vi "CT-Compute Max Level.vi"(0 "HCT Runtime":T3, 9 "Level":T1, 11 "error in (no error)":errorcluster) -> (6 "Max Level":dbl, 10 "Level out":T1, 15 "error out":errorcluster)   [LabVIEW 2020]
uses:
  CT-Runtime Data.ctl
  Controls/Level XCtl/Level Data.ctl
  Controls/Level XCtl/Level Units.ctl
  Utility VIs/Math VIs/Linear to dB (scalar).vi
  PXI DAQ VIs/DAQ Engine VIs/PXI Globals.vi
  Controls/Level XCtl/Level XCtl.xctl
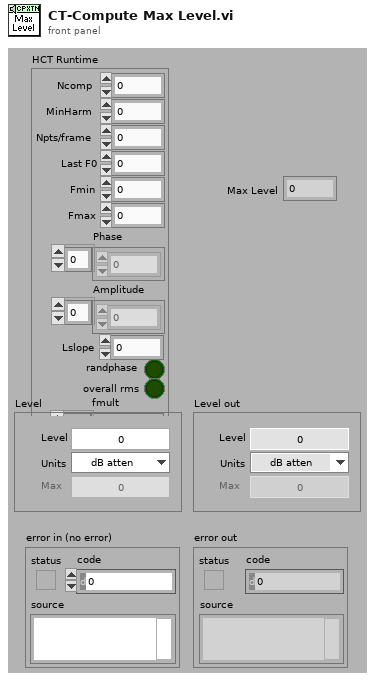
[diagram p1: front panel]
types:
  T1 = typedef "Level XCtl.xctl/Level Data.ctl" = cluster{"Level":dbl, "Units":T2, "Max":dbl, "Multiplier":dbl, "Cal File":path, "Cal":cluster{"Freq (Hz)":dbl[], "Mag (dB SPL)":dbl[], "Phase (deg)":dbl[]}}
  T2 = typedef "Level Units.ctl" = enum16{"dB atten", "dB SPL", "dB re 1 Vrms", "dB V/Hz½", "mW", "dB HL", "Volts", "dB mW"}
  T3 = typedef "CT-Runtime Data.ctl" = cluster{"Ncomp":i32, "MinHarm":i32, "Phase":dbl[], "Amplitude":dbl[], "Npts/frame":i32, "Last F0":dbl, "Fmin":dbl, "Fmax":dbl, "Lslope":dbl, "randphase":bool, "overall rms":bool, "fmult":dbl[], "jittered":bool}
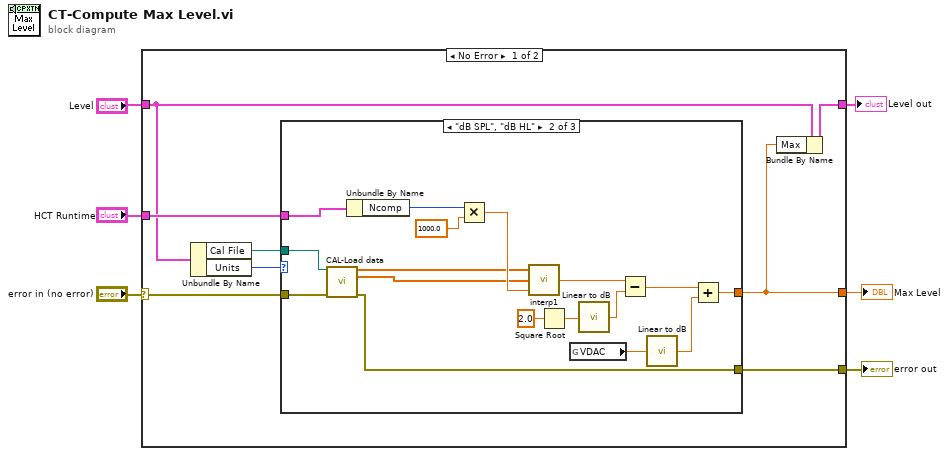
[diagram p0: block diagram]
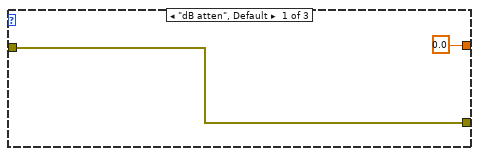
[diagram p2: hidden frame]
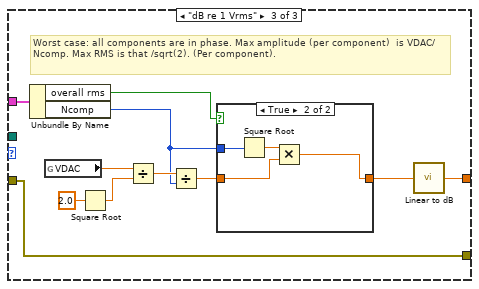
[diagram p3: hidden frame]
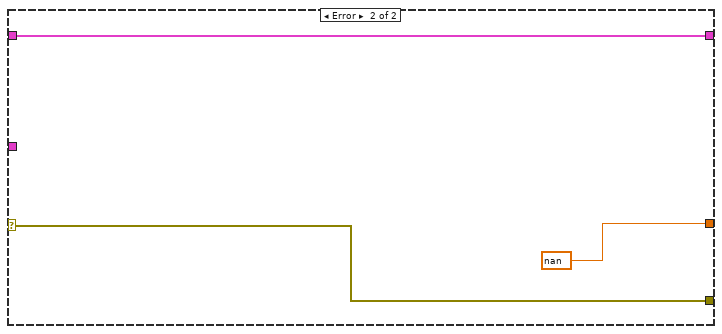
[diagram p5: hidden frame]
diagram:
  n1 = case shown="No Error" "error in (no error)" {
    selector: "error in (no error)" -> [w14 w52]
    tunnel: "Level" -> [w11 w50]
    tunnel: "HCT Runtime" -> [w13 _]
    tunnel: [w12 w52] -> w5
    tunnel: [w10 nan ("Reference Level")] -> w2
    tunnel: [w9 w50] -> w1
    frame No Error {
      n2 = Unbundle By Name(w11) -> ("Cal File"=w8:path, "Units"=w7:T2)
      n3 = case shown="\"dB SPL\", \"dB HL\"" w7 {
        tunnel: w14 -> [w15 w33 w44]
        tunnel: w13 -> [_ w24 w40]
        tunnel: [0.0 ("Reference Level") w31 w34] -> w10
        tunnel: [w15 w20 w44] -> w12
        tunnel: w8 -> [_ w19 _]
        frame "dB atten", Default {
        }
        frame "dB SPL", "dB HL" {
          n4 = call "CAL-Load data.vi"("user path"=w19, "error in (no error)"=w33) -> ("Frequency (Hz)"=w18:dbl[], "Mag"=w17:dbl[], "error out"=w20:errorcluster)  [unwired: 6 in, 5 out]
          n5 = Unbundle By Name(w24) -> ("Ncomp"=w29:i32)
          n6 = Multiply(x=w29, y=1000.0) -> (x*y=w27:dbl)
          n7 = call "interp1.vi"("X"=w18, "Y"=w17, "U"=w27) -> ("V"=w25:dbl)  [unwired: 2 in]
          n8 = Square Root(x=2.0 ("y")) -> (sqrt(x)=w23:dbl)
          n9 = global read "PXI Globals.vi" "VDAC"() -> (w32:dbl)
          n10 = call-poly "Linear to dB.vi"("Linear"=w23) -> ("dB"=w22:dbl)
          n11 = Subtract(x=w25, y=w22) -> (x-y=w21:dbl)
          n12 = call-poly "Linear to dB.vi"("Linear"=w32) -> ("dB"=w30:dbl)
          n13 = Add(x=w21, y=w30) -> (x+y=w31:dbl)
        }
        frame "dB re 1 Vrms" {
          # "Worst case: all components are in phase. Max amplitude (per component)  is VDAC/Ncomp. Max RMS is that /sqrt(2). (Per component)."
          n14 = Unbundle By Name(w40) -> ("overall rms"=w36:bool, "Ncomp"=w38:i32)
          n15 = global read "PXI Globals.vi" "VDAC"() -> (w41:dbl)
          n16 = Square Root(x=2.0 ("y")) -> (sqrt(x)=w42:dbl)
          n17 = Divide(x=w41, y=w42) -> (x/y=w39:dbl)
          n18 = Divide(x=w39, y=w38) -> (x/y=w35:dbl)
          n19 = case shown="True" w36 {
            tunnel: w38 -> [_ w49]
            tunnel: [w45 w46] -> w37
            tunnel: w35 -> [w45 w47]
            frame False {
            }
            frame True {
              n20 = Square Root(x=w49) -> (sqrt(x)=w48:dbl)
              n21 = Multiply(x=w48, y=w47) -> (x*y=w46:dbl)
            }
          }
          n22 = call-poly "Linear to dB.vi"("Linear"=w37) -> ("dB"=w34:dbl)
        }
      }
      n23 = Bundle By Name(cluster=w11, "Max"=w10) -> (w9:T1)
    }
    frame Error {
    }
  }
  "error out" <- w5
  "Max Level" <- w2
  "Level out" <- w1
